vi "Read Results.vi"(8 "error in (no error)":errorcluster, 11 "StellarNetSpecAcquisition in":refnum<class "StellarNetSpecAcquisition.lvclass">) -> (0 "error out":errorcluster, 2 "Results":T1, 3 "StellarNetSpecAcquisition out":refnum<class "StellarNetSpecAcquisition.lvclass">)   [LabVIEW 2020, in "StellarNetSpecAcquisition.lvclass"]
uses:
  StellarNetSpecAcquisition.lvclass
  StellarNetSpecAcquisition.lvclass/StellarNetSpecAcquisition.ctl
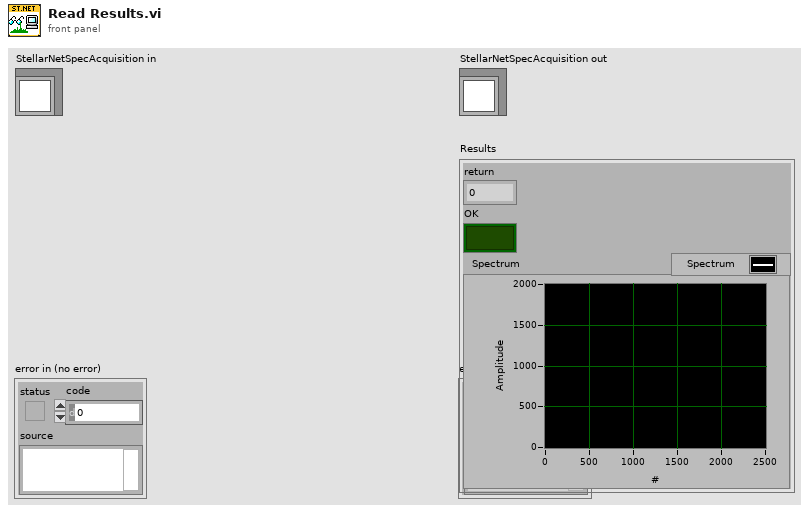
[diagram p1: front panel]
types:
  T1 = cluster{"return":i32, "OK":bool, "Spectrum":sgl[]}
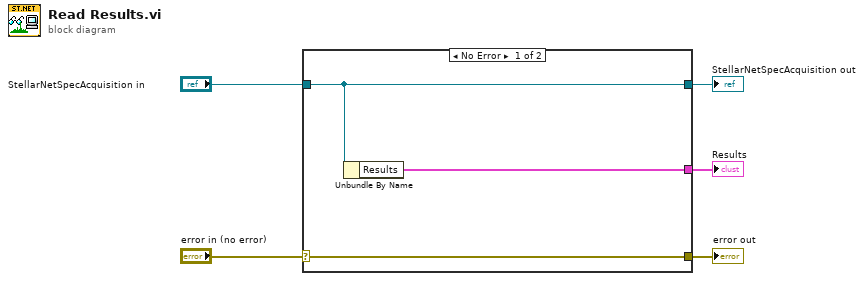
[diagram p0: block diagram]
diagram:
  n1 = case shown="No Error" "error in (no error)" {
    selector: "error in (no error)" -> [w8 w9]
    tunnel: [w8 w9] -> w4
    tunnel: [w7 w10] -> w2
    tunnel: "StellarNetSpecAcquisition in" -> [w7 w10]
    tunnel: [w6 _] -> w1
    frame No Error {
      n2 = Unbundle By Name(w7) -> ("Results"=w6:T1)
    }
    frame Error {
    }
  }
  "error out" <- w4
  "StellarNetSpecAcquisition out" <- w2
  "Results" <- w1
